vi "Configure Data Log Markers.vi"(8 "error in (no error)":errorcluster {"code" format="%.0x"}, 9 "Data Log Marker 2 (27.5 s)":dbl=27.5 format="%^.3e", 10 "Data Log Marker 1 (7.5 s)":dbl=7.5 format="%^.3e", 11 "VISA resource name":refnum<visa-resource-name>) -> (0 "error out":errorcluster {"code" format="%.0x"}, 3 "VISA resource name out":refnum<visa-resource-name>)   [LabVIEW 2018, in "Agilent N6700 Series.lvlib"]
doc: "Sets the position of the data logger markers. \n\n<b>Note:</b>\nThis VI only applies to the N6705B and N6705C DC Power Analyzer."
uses:
  Agilent N6700 Series.lvlib
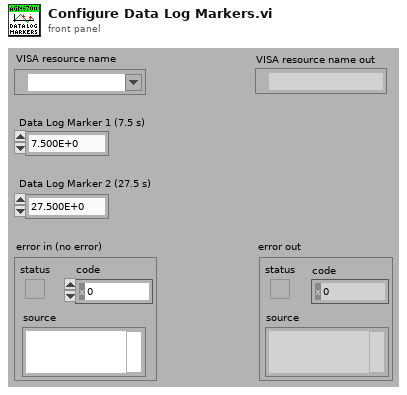
[diagram p1: front panel]
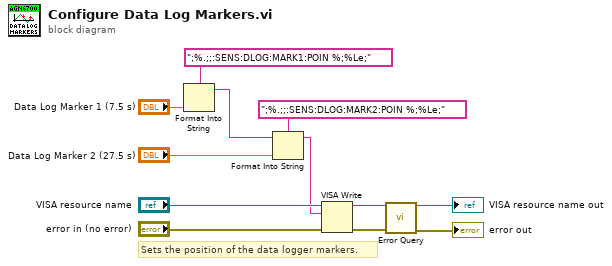
[diagram p0: block diagram]
diagram:
  # "Sets the position of the data logger markers."
  n1 = Format Into String(format string=";%.;;:SENS:DLOG:MARK1:POIN %;%Le;", "Data Log Marker 1 (7.5 s)") -> (resulting string=w5:string)  [unwired: 2 in, 1 out]
  n2 = Format Into String(format string=";%.;;:SENS:DLOG:MARK2:POIN %;%Le;", initial string=w5, "Data Log Marker 2 (27.5 s)") -> (resulting string=w1:string)  [unwired: 1 in, 1 out]
  n3 = VISA Write(VISA resource name="VISA resource name", write buffer=w1, error in (no error)="error in (no error)") -> (VISA resource name out=w8:refnum<visa-resource-name>, error out=w7:errorcluster)  [unwired: 1 out]
  n4 = call "Error Query.vi"("VISA resource name"=w8, "error in (no error)"=w7) -> ("VISA resource name out"=→"VISA resource name out":refnum<visa-resource-name>, "error out"=→"error out":errorcluster)  [unwired: 10 in, 2 out]
